vi "Autosize Build Menu.vi"(10 "Selection List[]":refnum<vi>[](array[refnum])) -> (2 "Menu":string)   [LabVIEW 2015]
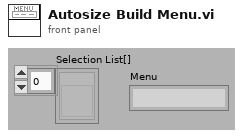
[diagram p1: front panel]
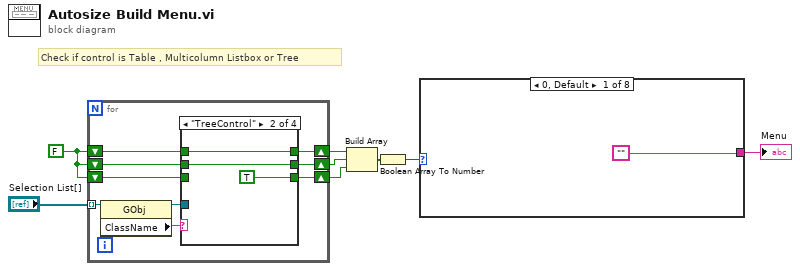
[diagram p0: block diagram]
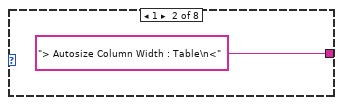
[diagram p2: hidden frame]
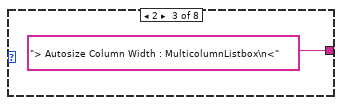
[diagram p3: hidden frame]
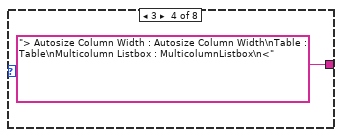
[diagram p4: hidden frame]
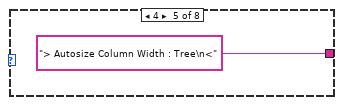
[diagram p5: hidden frame]
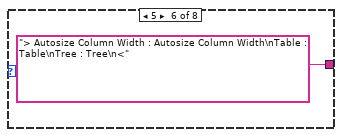
[diagram p6: hidden frame]
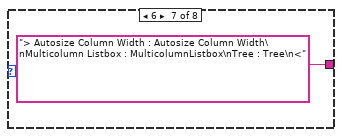
[diagram p7: hidden frame]
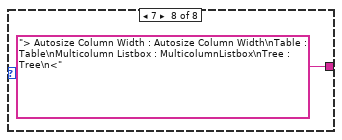
[diagram p8: hidden frame]
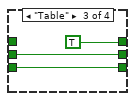
[diagram p10: hidden frame]
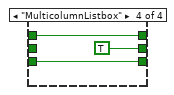
[diagram p11: hidden frame]
diagram:
  w4 = FALSE
  # "Check if control is Table , Multicolumn Listbox or Tree"
  n1 = for {
    tunnel: "Selection List[]" -> [w17] mode=indexing
    shift-right: [w14] -> w6
    shift-left: w4 -> [w13]
    shift-right: [w12] -> w5
    shift-left: w4 -> [w11]
    shift-right: [w9] -> w3
    shift-left: w4 -> [w10]
    n2 = property class="GObj"(reference=w17) -> (reference out=w15:refnum<vi>, "ClassName"=w16:string)  [unwired: 1 in, 1 out]
    n3 = case shown="\"TreeControl\"" w16 {
      tunnel: w15 -> [_ _ _ _]
      tunnel: [w20 w23 TRUE w29] -> w14
      tunnel: w13 -> [w20 w23 _ w29]
      tunnel: [w19 w22 w26 TRUE] -> w12
      tunnel: w11 -> [w19 w22 w26 _]
      tunnel: w10 -> [w18 _ w24 w27]
      tunnel: [w18 TRUE w24 w27] -> w9
      frame Default {
      }
      frame "TreeControl" {
      }
      frame "Table" {
      }
      frame "MulticolumnListbox" {
      }
    }
  }
  n4 = Build Array(w6, w5, w3) -> (w7:bool[])
  n5 = Boolean Array To Number(Boolean array=w7) -> (number=w2:u32)
  n6 = case shown="0, Default" w2 {
    tunnel: ["" "> Autosize Column Width : Table\n<" "> Autosize Column Width : MulticolumnListbox\n<" "> Autosize Column Width : Autosize Column Width\nTable : Table\nMulticolumn Listbox : MulticolumnListbox\n<" "> Autosize Column Width : Tree\n<" "> Autosize Column Width : Autosize Column Width\nTable : Table\nTree : Tree\n<" "> Autosize Column Width : Autosize Column Width\nMulticolumn Listbox : MulticolumnListbox\nTree : Tree\n<" "> Autosize Column Width : Autosize Column Width\nTable : Table\nMulticolumn Listbox : MulticolumnListbox\nTree : Tree\n<"] -> w1
    frame 0, Default {
    }
    frame 1 {
    }
    frame 2 {
    }
    frame 3 {
    }
    frame 4 {
    }
    frame 5 {
    }
    frame 6 {
    }
    frame 7 {
    }
  }
  "Menu" <- w1
